vi "FRIC_SerialPortOpen.vi"(0 "Baud Rate":u32=9600, 1 "Timeout Value (ms)":u32=5000, 2 "Termination Char (0xA = '\\n' = LF)":u8=10 format="%.0x", 3 "Enable Termination Char? (T)":bool=TRUE, 5 "Data Bits":u16=8, 7 "Parity":u16(ring) items=["None", "Odd", "Even", "Mark", "Space"], 9 "Stop Bits":u16(ring)=10 items=["1.0"=10, "1.5"=15, "2.0"=20], 11 "error in (no error)":errorcluster, 12 "Flow Control":u16(ring) items=["None", "XON/XOFF", "RTS/CTS", "XON/XOFF & RTS/CTS", "DTR/DSR", "XON/XOFF & DTR/DSR"], 13 "Serial Port":T1) -> (4 "SerialPortRef":T2, 15 "error out":errorcluster)   [LabVIEW 2016, in "navX Library.lvlib"]
doc: "Opens a reference to the serial port. You must open a reference before using any other VIs on this palette.\n\nThis software is licensed. Open the labview\\readme\\WPI Robotics Library Open Source License.txt file for more information."
uses:
  <vilib>/Rock Robotics/WPI/SerialPort/WPI_SerialPortRef.ctl
  <vilib>/Rock Robotics/WPI/SerialPort/WPI_SerialPort.ctl
  <vilib>/Instr/_visa.llb/VISA Open Access Mode.ctl
  <vilib>/Rock Robotics/SystemInterfaces/NetworkCommunication/NetComm_UsageReport_ResourceType.ctl
  <vilib>/Instr/_visa.llb/VISA Configure Serial Port (Instr).vi
  navX Library.lvlib
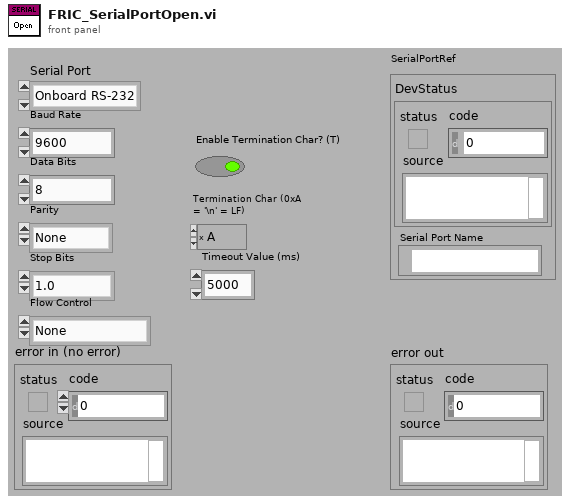
[diagram p1: front panel]
types:
  T1 = typedef "WPI_SerialPort.ctl" = enum16{"Onboard RS-232", "MXP TTL", "USB 1", "USB 2"}
  T2 = typedef "WPI_SerialPortRef.ctl" = cluster{"DevStatus":errorcluster, "Serial Port Name":refnum<visa-resource-name>}
  T3 = typedef "VISA Open Access Mode.ctl" = u32
  T4 = typedef "NetComm_UsageReport_ResourceType.ctl" = enum8{"Controller", "Module", "Language", "CANPlugin", "Accelerometer", "ADXL345", "AnalogChannel", "AnalogTrigger", "AnalogTriggerOutput", "CANJaguar", "Compressor", "Counter", "Dashboard", "DigitalInput", "DigitalOutput", "DriverStationCIO", "DriverStationEIO", "DriverStationLCD", "Encoder", "GearTooth", "Gyro", "I2C", "Framework", "Jaguar", "Joystick", "Kinect", "KinectStick", "PIDController", "Preferences", "PWM", "Relay", "RobotDrive", "SerialPort", "Servo", "Solenoid", "SPI", "Task", "Ultrasonic", "Victor", "Button", "Command", "AxisCamera", "PCVideoServer", "SmartDashboard", "Talon", "HiTechnicColorSensor", "HiTechnicAccel", "HiTechnicCompass", "SRF08", "AnalogOutput", "Victor SP", "Talon SRX", "CAN Talon SRX", "ADXL362 Accel", "ADXRS450 Gyro", "Rev SPARK", "Mindsensors SD540", "Digital Filter", "ADIS16448", "PDP", "PCM", "PigeonIMU"}
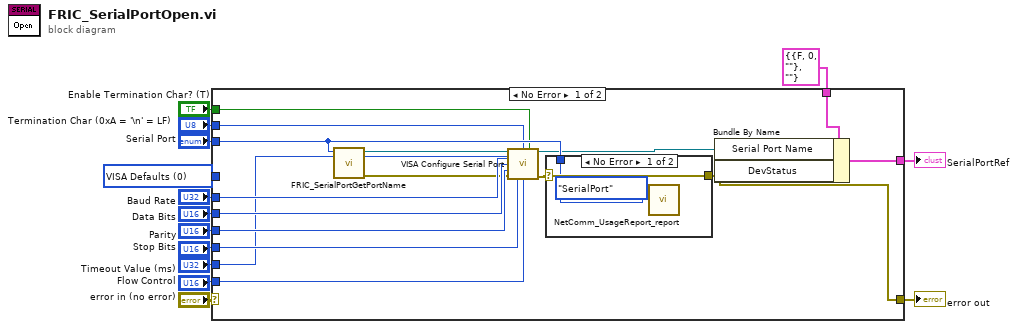
[diagram p0: block diagram]
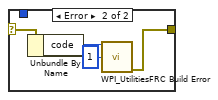
[diagram p2: hidden frame]
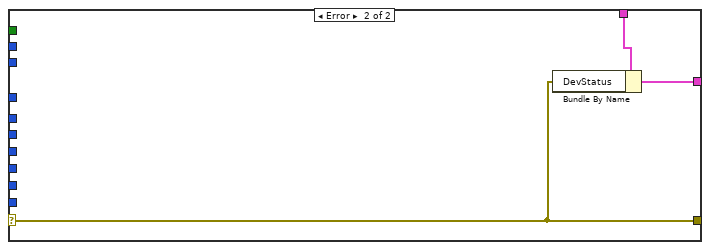
[diagram p3: hidden frame]
diagram:
  w1 = T3 0 items=["VISA Defaults"=0, "Exclusive Lock"=1, "Load Configured Settings"=4] ("Access Mode")
  n1 = case shown="No Error" "error in (no error)" {
    selector: "error in (no error)" -> [_ w39]
    tunnel: "Baud Rate" -> [w27 _]
    tunnel: "Parity" -> [w25 _]
    tunnel: "Data Bits" -> [w26 _]
    tunnel: [w20 w40] -> w11
    tunnel: "Stop Bits" -> [w24 _]
    tunnel: [w19 w39] -> w8
    tunnel: T2 {"DevStatus"={"status"=FALSE, "code"=0, "source"=""}, "Serial Port Name"=""} ("SerialPortRef") -> [w30 w38]
    tunnel: "Enable Termination Char? (T)" -> [w17 _]
    tunnel: "Termination Char (0xA = '\\n' = LF)" -> [w21 _]
    tunnel: "Timeout Value (ms)" -> [w22 _]
    tunnel: "Flow Control" -> [w23 _]
    tunnel: "Serial Port" -> [w29 _]
    tunnel: w1 -> [_ _]
    frame No Error {
      n2 = call "FRIC_SerialPortGetPortName.vi"("Serial Port"=w29) -> ("error out"=w16:errorcluster, "VISA Refnum out"=w15:refnum<visa-resource-name>)  [unwired: 9 in]
      n3 = call-poly "VISA Configure Serial Port"("VISA resource name"=w15, "timeout (10sec)"=w22, "termination char\n(0xA = '\\n' = LF)"=w21, "Enable Termination\nChar (T)"=w17, "baud rate (9600)"=w27, "data bits (8)"=w26, "parity (0:none)"=w25, "error in (no error)"=w16, "stop bits (10: 1 bit)"=w24, "flow control (0:none)"=w23) -> ("VISA resource name out"=w28:refnum<visa-resource-name>, "error out"=w18:errorcluster)  [unwired: 4 in]
      n4 = case shown="No Error" w18 {
        selector: w18 -> [w33 w35]
        tunnel: [w33 w34] -> w19
        tunnel: w29 -> [w31 _]
        frame No Error {
          n5 = call <vilib>:"NetComm_UsageReport_report.vi"("Instance Number"=w31, "Resource Type"=NetComm_UsageReport_ResourceType."SerialPort") -> ()  [unwired: 10 in]
        }
        frame Error {
          n6 = Unbundle By Name(w35) -> ("code"=w37:i32)
          n7 = call <vilib>:"WPI_UtilitiesFRC Build Error.vi"("error code"=w37, "chain levels to remove (1)"=1) -> ("error out"=w34:errorcluster)  [unwired: 3 in, 10 out]
        }
      }
      n8 = Bundle By Name(cluster=w30, "Serial Port Name"=w28, "DevStatus"=w19) -> (w20:T2)
    }
    frame Error {
      n9 = Bundle By Name(cluster=w38, "DevStatus"=w39) -> (w40:T2)
    }
  }
  "error out" <- w8
  "SerialPortRef" <- w11
